vi "Write to Port.vi"(10 "value":i16, 11 "AO in":refnum<class "Analog Output.lvclass">) -> ()   [LabVIEW 2017, in "Analog IO.lvlib" / "Analog Output.lvclass"]
uses:
  Analog Output.lvclass
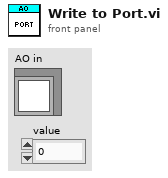
[diagram p1: front panel]
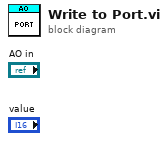
[diagram p0: block diagram]
diagram:
